vi "PicoScope6000GetBlock.vi"(0 "error in":errorcluster, 2 "handle in":i16, 3 "Acquisition Settings":T3 {"Down Sample Ratio" min=1 step=1; "Down-Sample Mode" items=["None", "Aggregate", "Average", "Decimate", "Distribution"]}, 8 "Enabled array":i16[](array[numeric])) -> (1 "noOfSamples":u32, 4 "overflow":i16, 6 "error out":errorcluster, 7 "handle out":i16, 9 "Buffers (Max or non-aggregated)":T1, 10 "Min Buffers":T2)   [LabVIEW 2009]
doc: "This VI collects a block of data from the oscilloscope. This can be called in a loop in order to continually collect blocks of data. The oscilloscope should first be set up by using PicoScope6000Settings.vi. The VI outputs data arrays in two clusters (max and min). If not using aggregation, 'Min Buffers' is not used."
uses:
  PS6000.dll
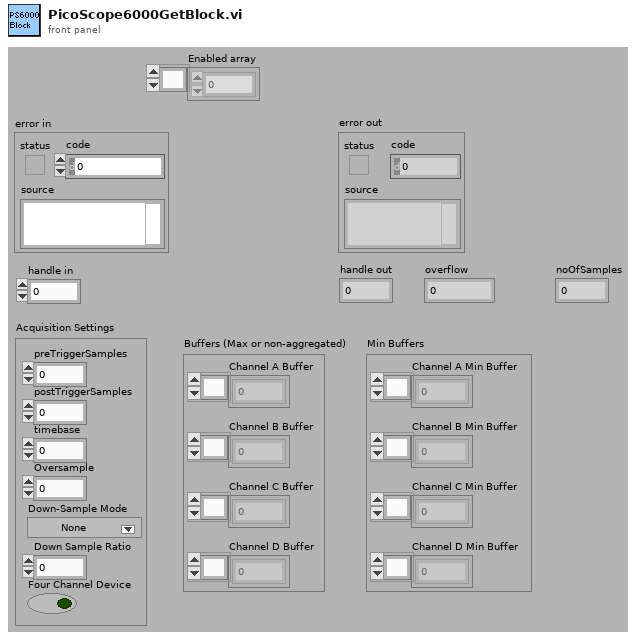
[diagram p1: front panel]
types:
  T1 = cluster{"Channel D Buffer":i16[], "Channel C Buffer":i16[], "Channel B Buffer":i16[], "Channel A Buffer":i16[]}
  T2 = cluster{"Channel A Min Buffer":i16[], "Channel B Min Buffer":i16[], "Channel C Min Buffer":i16[], "Channel D Min Buffer":i16[]}
  T3 = cluster{"preTriggerSamples":u32, "postTriggerSamples":u32, "timebase":u32, "Down-Sample Mode":i32, "Down Sample Ratio":u32, "Four Channel Device":bool, "Oversample":i16}
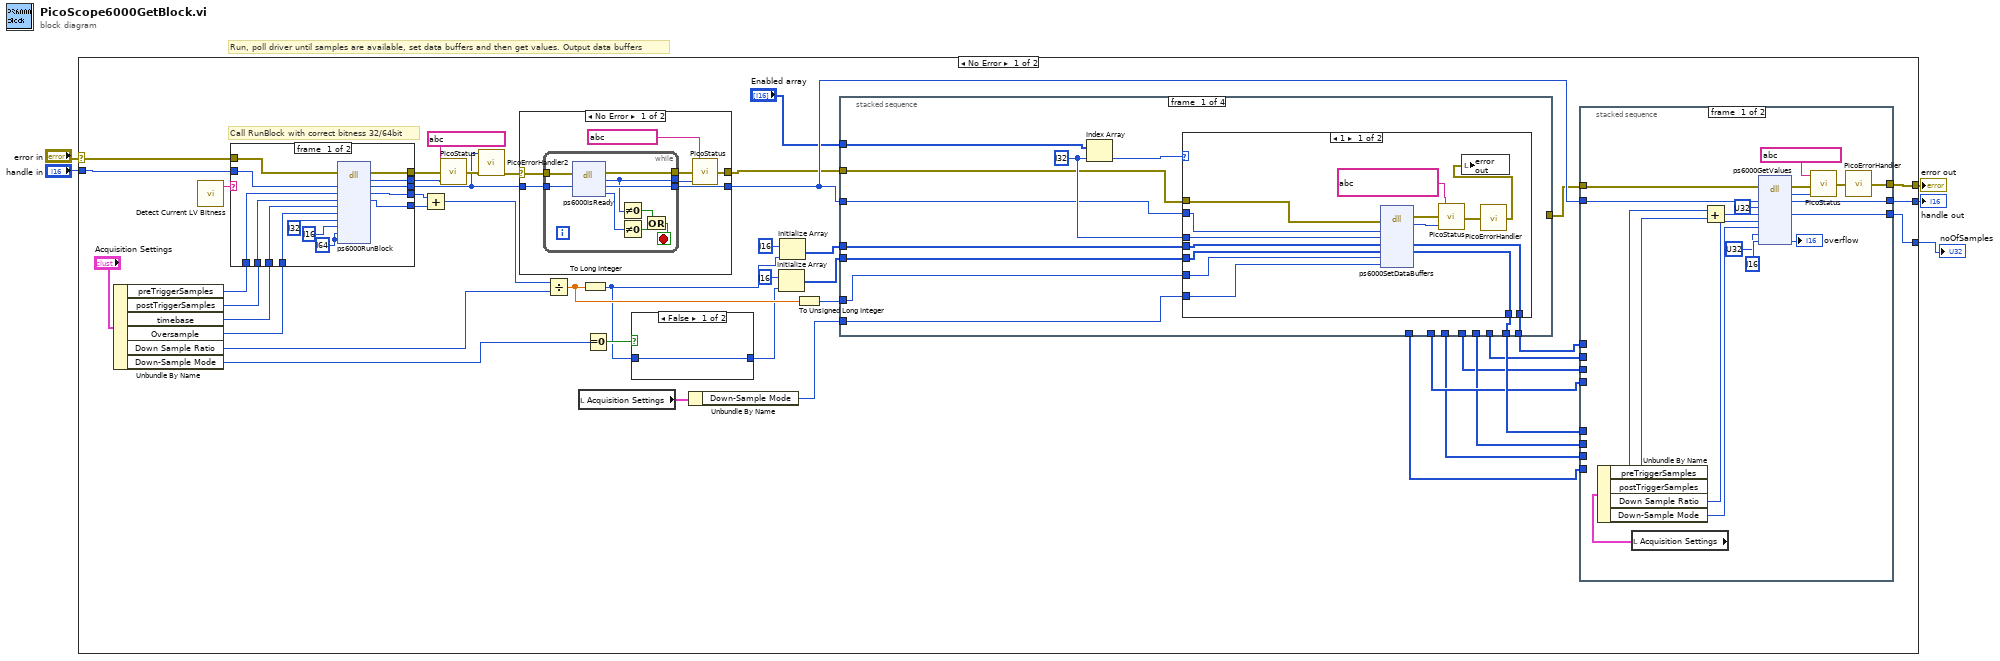
[diagram p0: block diagram]
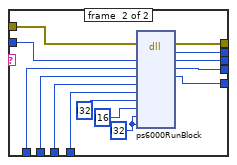
[diagram p2: hidden frame]
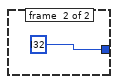
[diagram p3: hidden frame]
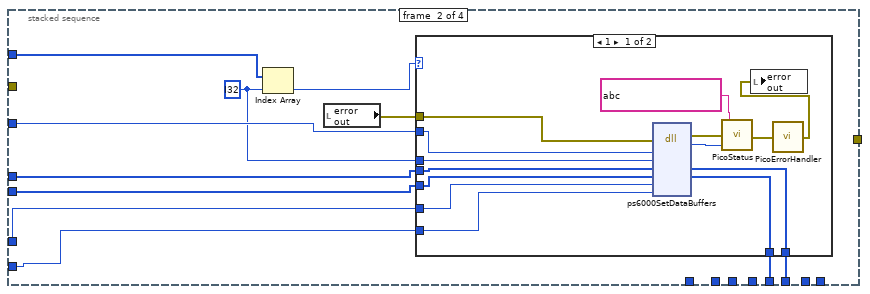
[diagram p5: hidden frame]
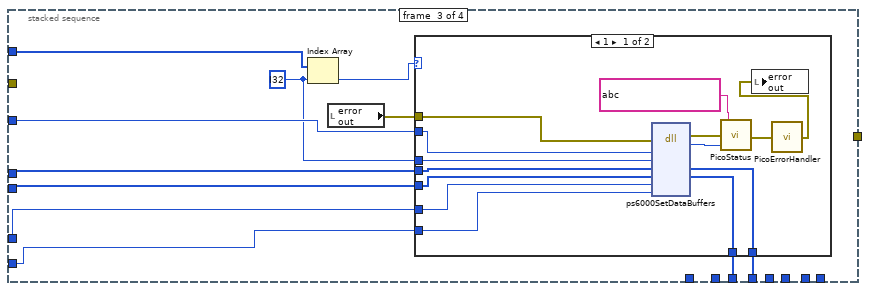
[diagram p7: hidden frame]
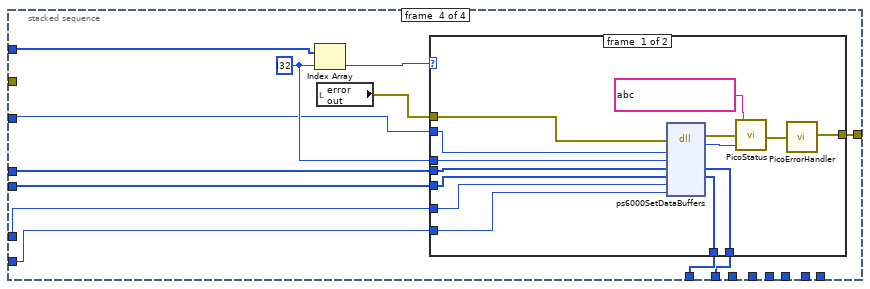
[diagram p9: hidden frame]
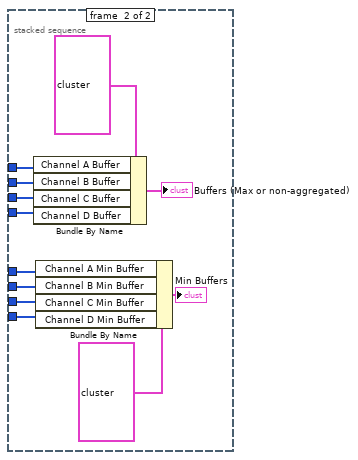
[diagram p11: hidden frame]
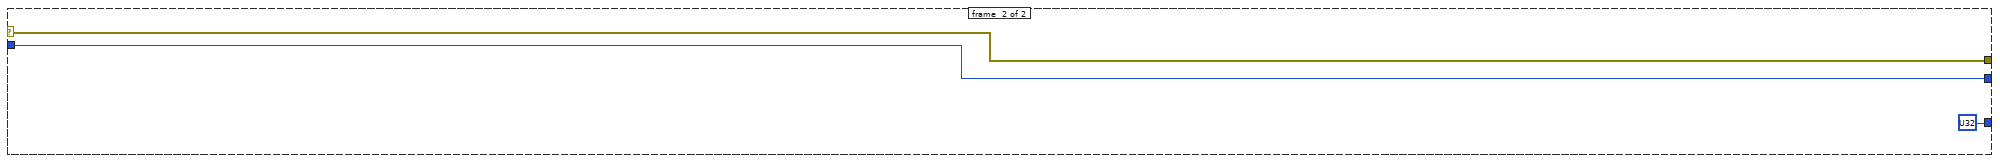
[diagram p13: hidden frame]
diagram:
  # "Run, poll driver until samples are available, set data buffers and then get values. Output data buffers"
  n1 = case shown="No Error" "error in" {
    selector: "error in" -> [w41 w234]
    tunnel: [w42 w234] -> w4
    tunnel: "handle in" -> [w40 w233]
    tunnel: [w39 w233] -> w2
    tunnel: [w13 u32 ? ("noOfSamples")] -> w1
    frame #0 {
      # "Call RunBlock with correct bitness 32/64bit"
      n2 = Unbundle By Name("Acquisition Settings") -> ("preTriggerSamples"=w47:u32, "postTriggerSamples"=w46:u32, "timebase"=w48:u32, "Oversample"=w36:i16, "Down Sample Ratio"=w37:u32, "Down-Sample Mode"=w16:i32)
      n3 = call "Detect Current LV Bitness.vi"() -> ("bitness"=w9:string)  [unwired: 11 in]
      n4 = case shown="\"32\", Default" w9 {
        tunnel: w48 -> [w64 w78]
        tunnel: w47 -> [w63 w77]
        tunnel: w46 -> [w62 w76]
        tunnel: [w61 w75] -> w45
        tunnel: [w60 w74] -> w44
        tunnel: w41 -> [w59 w73]
        tunnel: w40 -> [w58 w72]
        tunnel: w36 -> [w57 w71]
        tunnel: [w56 w70] -> w10
        tunnel: [w52 w66] -> w8
        tunnel: [w51 w65] -> w7
        frame #0 {
          w54 = i64 ? ("pParameter")
          n5 = dll-call lib="PS6000.dll" fn="ps6000RunBlock" ("ps3000.dll:_ps3000_open_unit@0")(error in=w59, "handle"=w58, "preTriggerSamples"=w63, "postTriggerSamples"=w62, "timebase"=w64, "oversample"=w57, "timeindisposed"=i32 ? ("pParameter"), "segmentIndex"=i16 ? ("pParameter"), "lpReady"=w54, "pParameter"=w54) -> (error out=w60:errorcluster, "PICO_STATUS"=w61:u32, "handle"=w56:i16, "preTriggerSamples"=w51:u32, "postTriggerSamples"=w52:u32)  [unwired: 8 in, 1 out]
        }
        frame #1 {
          w68 = i32 ? ("pParameter")
          n6 = dll-call lib="PS6000.dll" fn="ps6000RunBlock" ("ps3000.dll:_ps3000_open_unit@0")(error in=w73, "handle"=w72, "preTriggerSamples"=w77, "postTriggerSamples"=w76, "timebase"=w78, "oversample"=w71, "timeindisposed"=i32 ? ("pParameter"), "segmentIndex"=i16 ? ("pParameter"), "lpReady"=w68, "pParameter"=w68) -> (error out=w74:errorcluster, "PICO_STATUS"=w75:u32, "handle"=w70:i16, "preTriggerSamples"=w65:u32, "postTriggerSamples"=w66:u32)  [unwired: 8 in, 1 out]
        }
      }
      n7 = Add(x=w7, y=w8) -> (x+y=w6:u32)
      n8 = call "PicoStatus.vi"("PICO STATUS"=w45, "error in"=w44, "source"=string ?) -> ("error out"=w11:errorcluster)
      n9 = call "PicoErrorHandler2.vi"("error in (no error)"=w11, "handle In"=w10) -> ("error out"=w12:errorcluster)  [unwired: 9 in]
      n10 = case shown="No Error" w12 {
        selector: w12 -> [w218 w230]
        tunnel: w10 -> [w220 w231]
        tunnel: [w219 w231] -> w33
        tunnel: [w217 w230] -> w31
        frame #0 {
          n11 = while {
            tunnel: [w229] -> w219
            tunnel: w220 -> [w228]
            tunnel: [w223] -> w215
            tunnel: w218 -> [w222]
            tunnel: [w221] -> w216
            stop <- w227 stop-if-true
            n12 = dll-call lib="PS6000.dll" fn="ps6000IsReady" ("ps3000.dll:_ps3000_open_unit@0")(error in=w222, "handle"=w228) -> (error out=w221:errorcluster, "status"=w223:u32, "handle"=w229:i16, "ready"=w224:i16)  [unwired: 3 in, 1 out]
            n13 = Not Equal To 0?(x=w223) -> (x != 0?=w225:bool)
            n14 = Not Equal To 0?(x=w224) -> (x != 0?=w226:bool)
            n15 = Or(x=w225, y=w226) -> (x .or. y?=w227:bool)
          }
          n16 = call "PicoStatus.vi"("PICO STATUS"=w215, "error in"=w216, "source"=string ?) -> ("error out"=w217:errorcluster)
        }
        frame #1 {
        }
      }
      n17 = Divide(x=w6, y=w37) -> (x/y=w19:dbl)
      n18 = local read "Acquisition Settings"() -> (w27:T3)
      n19 = To Long Integer(number=w19) -> (32bit integer=w14:i32)
      n20 = Equal To 0?(x=w16) -> (x = 0?=w17:bool)
      n21 = case shown="False" w17 {
        tunnel: [w79 i32 ?] -> w15
        tunnel: w14 -> [w79 _]
        frame #0 {
        }
        frame #1 {
        }
      }
      n22 = Unbundle By Name(w27) -> ("Down-Sample Mode"=w32:i32)
      n23 = Initialize Array(i16 ? ("element"), w15) -> (w29:i16[])
      n24 = Initialize Array(i16 ? ("element"), w14) -> (w30:i16[])
      n25 = To Unsigned Long Integer(number=w19) -> (unsigned 32bit integer=w18:u32)
      n26 = stacked-sequence {
        tunnel: [w90 _ _ _] -> w35
        tunnel: [w89 _ _ _] -> w34
        tunnel: w33 -> [w87 w113 w135 w164]
        tunnel: w32 -> [w86 w111 w138 w161]
        tunnel: w31 -> [w85 _ _ _]
        tunnel: w30 -> [w84 w110 w136 w163]
        tunnel: w29 -> [w83 w109 w137 w162]
        tunnel: "Enabled array" -> [w82 w114 w139 w165]
        tunnel: [_ _ _ w159] -> w26
        tunnel: [_ _ _ w157] -> w25
        tunnel: [_ _ _ w158] -> w24
        tunnel: [_ w108 _ _] -> w23
        tunnel: [_ w107 _ _] -> w22
        tunnel: [_ _ w133 _] -> w21
        tunnel: [_ _ w132 _] -> w20
        tunnel: w18 -> [w81 w106 w131 w156]
        frame #0 {
          w88 = i32 ? ("dimension size")
          n27 = Index Array(array=w82, index=w88) -> (element=w91:i16)
          n28 = case shown="1" w91 {
            tunnel: [w101 _] -> w90
            tunnel: [w100 _] -> w89
            tunnel: w85 -> [w99 _]
            tunnel: w88 -> [w98 _]
            tunnel: w87 -> [w97 _]
            tunnel: w86 -> [w96 _]
            tunnel: w84 -> [w95 _]
            tunnel: w83 -> [w94 _]
            tunnel: w81 -> [w92 _]
            frame #0 {
              n29 = dll-call lib="PS6000.dll" fn="ps6000SetDataBuffers" ("ps3000.dll:_ps3000_open_unit@0")(error in=w99, "handle"=w97, "channel"=w98, "bufferMax"=w95, "bufferMin"=w94, "bufferLth"=w92, "downSampleRatioMode"=w96) -> (error out=w104:errorcluster, "PICO_STATUS"=w105:u32, "bufferMax"=w101:i16[], "bufferMin"=w100:i16[])  [unwired: 6 in, 1 out]
              n30 = call "PicoStatus.vi"("PICO STATUS"=w105, "error in"=w104, "source"=string ?) -> ("error out"=w102:errorcluster)
              n31 = call "PicoErrorHandler.vi"("error in"=w102) -> ("error out"=w93:errorcluster)
              n32 = local write "error out"(w93) -> ()
            }
            frame #1 {
            }
          }
        }
        frame #1 {
          w112 = i32 ? ("dimension size")
          n33 = Index Array(array=w114, index=w112) -> (element=w115:i16)
          n34 = local read "error out"() -> (w116:errorcluster)
          n35 = case shown="1" w115 {
            tunnel: [w126 _] -> w108
            tunnel: [w125 _] -> w107
            tunnel: w116 -> [w124 _]
            tunnel: w112 -> [w123 _]
            tunnel: w113 -> [w122 _]
            tunnel: w111 -> [w121 _]
            tunnel: w110 -> [w120 _]
            tunnel: w109 -> [w119 _]
            tunnel: w106 -> [w117 _]
            frame #0 {
              n36 = dll-call lib="PS6000.dll" fn="ps6000SetDataBuffers" ("ps3000.dll:_ps3000_open_unit@0")(error in=w124, "handle"=w122, "channel"=w123, "bufferMax"=w120, "bufferMin"=w119, "bufferLth"=w117, "downSampleRatioMode"=w121) -> (error out=w129:errorcluster, "PICO_STATUS"=w130:u32, "bufferMax"=w126:i16[], "bufferMin"=w125:i16[])  [unwired: 6 in, 1 out]
              n37 = call "PicoStatus.vi"("PICO STATUS"=w130, "error in"=w129, "source"=string ?) -> ("error out"=w127:errorcluster)
              n38 = call "PicoErrorHandler.vi"("error in"=w127) -> ("error out"=w118:errorcluster)
              n39 = local write "error out"(w118) -> ()
            }
            frame #1 {
            }
          }
        }
        frame #2 {
          w134 = i32 ? ("dimension size")
          n40 = Index Array(array=w139, index=w134) -> (element=w140:i16)
          n41 = local read "error out"() -> (w141:errorcluster)
          n42 = case shown="1" w140 {
            tunnel: [w151 _] -> w133
            tunnel: [w150 _] -> w132
            tunnel: w141 -> [w149 _]
            tunnel: w134 -> [w148 _]
            tunnel: w135 -> [w147 _]
            tunnel: w138 -> [w146 _]
            tunnel: w136 -> [w145 _]
            tunnel: w137 -> [w144 _]
            tunnel: w131 -> [w142 _]
            frame #0 {
              n43 = dll-call lib="PS6000.dll" fn="ps6000SetDataBuffers" ("ps3000.dll:_ps3000_open_unit@0")(error in=w149, "handle"=w147, "channel"=w148, "bufferMax"=w145, "bufferMin"=w144, "bufferLth"=w142, "downSampleRatioMode"=w146) -> (error out=w154:errorcluster, "PICO_STATUS"=w155:u32, "bufferMax"=w151:i16[], "bufferMin"=w150:i16[])  [unwired: 6 in, 1 out]
              n44 = call "PicoStatus.vi"("PICO STATUS"=w155, "error in"=w154, "source"=string ?) -> ("error out"=w152:errorcluster)
              n45 = call "PicoErrorHandler.vi"("error in"=w152) -> ("error out"=w143:errorcluster)
              n46 = local write "error out"(w143) -> ()
            }
            frame #1 {
            }
          }
        }
        frame #3 {
          w166 = i32 ? ("dimension size")
          n47 = Index Array(array=w165, index=w166) -> (element=w167:i16)
          n48 = local read "error out"() -> (w160:errorcluster)
          n49 = case shown="0, Default" w167 {
            tunnel: [w178 w182] -> w159
            tunnel: [w176 _] -> w157
            tunnel: [w175 _] -> w158
            tunnel: w160 -> [w174 w182]
            tunnel: w166 -> [w173 _]
            tunnel: w164 -> [w172 _]
            tunnel: w161 -> [w171 _]
            tunnel: w163 -> [w170 _]
            tunnel: w162 -> [w169 _]
            tunnel: w156 -> [w168 _]
            frame #0 {
              n50 = dll-call lib="PS6000.dll" fn="ps6000SetDataBuffers" ("ps3000.dll:_ps3000_open_unit@0")(error in=w174, "handle"=w172, "channel"=w173, "bufferMax"=w170, "bufferMin"=w169, "bufferLth"=w168, "downSampleRatioMode"=w171) -> (error out=w180:errorcluster, "PICO_STATUS"=w181:u32, "bufferMax"=w176:i16[], "bufferMin"=w175:i16[])  [unwired: 6 in, 1 out]
              n51 = call "PicoStatus.vi"("PICO STATUS"=w181, "error in"=w180, "source"=string ?) -> ("error out"=w177:errorcluster)
              n52 = call "PicoErrorHandler.vi"("error in"=w177) -> ("error out"=w178:errorcluster)
            }
            frame #1 {
            }
          }
        }
      }
      n53 = stacked-sequence {
        tunnel: w33 -> [w201 _]
        tunnel: w26 -> [w198 _]
        tunnel: [w193 _] -> w42
        tunnel: [w192 _] -> w39
        tunnel: w35 -> [_ w211]
        tunnel: w23 -> [_ w210]
        tunnel: w21 -> [_ w209]
        tunnel: w25 -> [_ w208]
        tunnel: w34 -> [_ w205]
        tunnel: w22 -> [_ w204]
        tunnel: w20 -> [_ w203]
        tunnel: w24 -> [_ w202]
        tunnel: [w183 _] -> w13
        frame #0 {
          n54 = local read "Acquisition Settings"() -> (w190:T3)
          n55 = Unbundle By Name(w190) -> ("preTriggerSamples"=w187:u32, "postTriggerSamples"=w188:u32, "Down Sample Ratio"=w189:u32, "Down-Sample Mode"=w185:i32)
          n56 = Add(x=w187, y=w188) -> (x+y=w186:u32)
          n57 = dll-call lib="PS6000.dll" fn="ps6000GetValues" ("ps3000.dll:_ps3000_open_unit@0")(error in=w198, "handle"=w201, "startIndex"=u32 ?, "noOfSamples"=w186, "downSampleRatio"=w189, "downSampleRatioMode"=w185, "segmentIndex"=u32 ?, "overflow"=i16 ?) -> (error out=w196:errorcluster, "PICO_STATUS"=w197:u32, "handle"=w192:i16, "noOfSamples"=w183:u32, "overflow"=→"overflow":i16)  [unwired: 6 in, 1 out]
          n58 = call "PicoStatus.vi"("PICO STATUS"=w197, "error in"=w196, "source"=string ?) -> ("error out"=w194:errorcluster)
          n59 = call "PicoErrorHandler.vi"("error in"=w194) -> ("error out"=w193:errorcluster)
        }
        frame #1 {
          n60 = Bundle By Name(cluster=T1 ? ("Buffers (Max or non-aggregated)"), "Channel A Buffer"=w211, "Channel B Buffer"=w210, "Channel C Buffer"=w209, "Channel D Buffer"=w208) -> (→"Buffers (Max or non-aggregated)":T1)
          n61 = Bundle By Name(cluster=T2 ? ("Min Buffers"), "Channel A Min Buffer"=w205, "Channel B Min Buffer"=w204, "Channel C Min Buffer"=w203, "Channel D Min Buffer"=w202) -> (→"Min Buffers":T2)
        }
      }
    }
    frame #1 {
    }
  }
  "error out" <- w4
  "handle out" <- w2
  "noOfSamples" <- w1
